vi "test Unsigned Integer Data Integrity.vi"(8 "error in (no error)":errorcluster, 11 "Data Manipulation Tests in":refnum<class "Data Manipulation Tests.lvclass">) -> (0 "error out":errorcluster, 3 "Data Manipulation Tests out":refnum<class "Data Manipulation Tests.lvclass">)   [LabVIEW 2017, in "Memory Manager Tests.lvlib" / "Data Manipulation Tests.lvclass"]
uses:
  Data Manipulation Tests.lvclass
  Source/Classes/Pointer/Write U8.vi
  Source/Classes/Pointer/Write U16.vi
  Source/Classes/Pointer/Write U32.vi
  Source/Classes/Pointer/Write U64.vi
  Source/Classes/Pointer/Write 1D U8.vi
  Source/Classes/Pointer/Write 1D U16.vi
  Source/Classes/Pointer/Write 1D U32.vi
  Source/Classes/Pointer/Write 1D U64.vi
  Source/Classes/Pointer/Pointer.lvclass
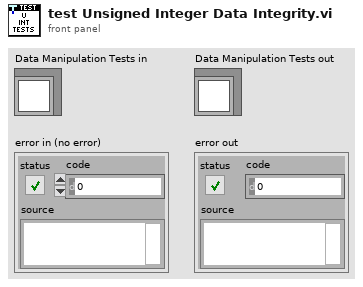
[diagram p1: front panel]
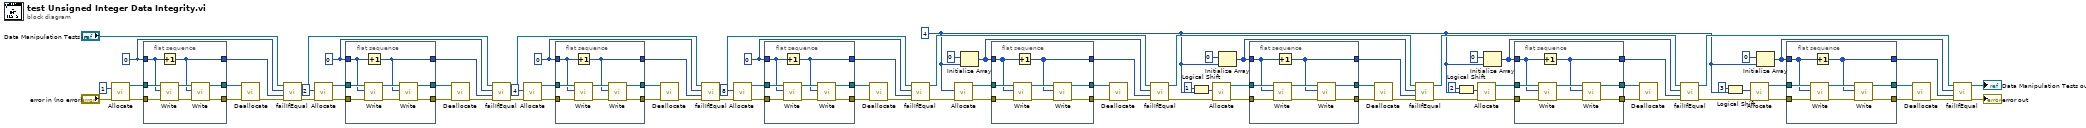
[diagram p0: block diagram]
diagram:
  w2 = u64 4 ("count (1)")
  w74 = u64 0 ("value")
  w84 = u32 0 ("value")
  w67 = u16 0 ("value")
  w56 = u8 0 ("value")
  n1 = call "Allocate.vi"("error in (no error)"="error in (no error)", "size"=u64 1) -> ("error out"=w58:errorcluster, "Pointer out"=w61:refnum<class "Pointer.lvclass">)  [unwired: 8 in]
  n2 = flat-sequence {
    tunnel: w61 -> [w97]
    tunnel: [w95] -> w60
    tunnel: [w94] -> w59
    tunnel: w58 -> [w92]
    tunnel: w56 -> [w91]
    tunnel: [w90] -> w55
    frame #0 {
      n3 = Increment(x=w91) -> (x+1=w90:u8)
      n4 = call-poly "Write.vi"("error in (no error)"=w92, "value"=w91, "Pointer in"=w97) -> ("error out"=w93:errorcluster, "Pointer out"=w96:refnum<class "Pointer.lvclass">)  [unwired: 5 in, 2 out]
      n5 = call-poly "Write.vi"("error in (no error)"=w93, "value"=w90, "Pointer in"=w96) -> ("error out"=w94:errorcluster, "Pointer out"=w95:refnum<class "Pointer.lvclass">)  [unwired: 5 in, 2 out]
    }
  }
  n6 = call "Deallocate.vi"("error in (no error)"=w59, "Pointer"=w60) -> ("error out"=w57:errorcluster)  [unwired: 8 in, 1 out]
  n7 = call-dynamic "failIfEqual.vi"("error in (no error)"=w57, "y"=w55, "x"=w56, "TestCase in"="Data Manipulation Tests in") -> ("error out"=w70:errorcluster, "TestCase out"=w69:refnum<class "Data Manipulation Tests.lvclass">)  [unwired: 6 in]
  n8 = call "Allocate.vi"("error in (no error)"=w70, "size"=u64 2) -> ("error out"=w65:errorcluster, "Pointer out"=w62:refnum<class "Pointer.lvclass">)  [unwired: 8 in]
  n9 = flat-sequence {
    tunnel: w62 -> [w105]
    tunnel: [w103] -> w63
    tunnel: [w102] -> w64
    tunnel: w65 -> [w100]
    tunnel: w67 -> [w99]
    tunnel: [w98] -> w68
    frame #0 {
      n10 = call-poly "Write.vi"("error in (no error)"=w100, "value"=w99, "Pointer in"=w105) -> ("error out"=w101:errorcluster, "Pointer out"=w104:refnum<class "Pointer.lvclass">)  [unwired: 5 in, 2 out]
      n11 = Increment(x=w99) -> (x+1=w98:u16)
      n12 = call-poly "Write.vi"("error in (no error)"=w101, "value"=w98, "Pointer in"=w104) -> ("error out"=w102:errorcluster, "Pointer out"=w103:refnum<class "Pointer.lvclass">)  [unwired: 5 in, 2 out]
    }
  }
  n13 = call "Deallocate.vi"("error in (no error)"=w64, "Pointer"=w63) -> ("error out"=w66:errorcluster)  [unwired: 8 in, 1 out]
  n14 = call-dynamic "failIfEqual.vi"("error in (no error)"=w66, "y"=w68, "x"=w67, "TestCase in"=w69) -> ("error out"=w87:errorcluster, "TestCase out"=w86:refnum<class "Data Manipulation Tests.lvclass">)  [unwired: 6 in]
  n15 = call "Allocate.vi"("error in (no error)"=w87, "size"=u64 4) -> ("error out"=w83:errorcluster, "Pointer out"=w80:refnum<class "Pointer.lvclass">)  [unwired: 8 in]
  n16 = flat-sequence {
    tunnel: w80 -> [w113]
    tunnel: [w111] -> w81
    tunnel: [w110] -> w82
    tunnel: w83 -> [w108]
    tunnel: w84 -> [w107]
    tunnel: [w106] -> w85
    frame #0 {
      n17 = call-poly "Write.vi"("error in (no error)"=w108, "value"=w107, "Pointer in"=w113) -> ("error out"=w109:errorcluster, "Pointer out"=w112:refnum<class "Pointer.lvclass">)  [unwired: 5 in, 2 out]
      n18 = Increment(x=w107) -> (x+1=w106:u32)
      n19 = call-poly "Write.vi"("error in (no error)"=w109, "value"=w106, "Pointer in"=w112) -> ("error out"=w110:errorcluster, "Pointer out"=w111:refnum<class "Pointer.lvclass">)  [unwired: 5 in, 2 out]
    }
  }
  n20 = call "Deallocate.vi"("error in (no error)"=w82, "Pointer"=w81) -> ("error out"=w9:errorcluster)  [unwired: 8 in, 1 out]
  n21 = call-dynamic "failIfEqual.vi"("error in (no error)"=w9, "y"=w85, "x"=w84, "TestCase in"=w86) -> ("error out"=w71:errorcluster, "TestCase out"=w72:refnum<class "Data Manipulation Tests.lvclass">)  [unwired: 6 in]
  n22 = call "Allocate.vi"("error in (no error)"=w71, "size"=u64 8) -> ("error out"=w76:errorcluster, "Pointer out"=w79:refnum<class "Pointer.lvclass">)  [unwired: 8 in]
  n23 = flat-sequence {
    tunnel: w79 -> [w121]
    tunnel: [w119] -> w78
    tunnel: [w118] -> w77
    tunnel: w76 -> [w116]
    tunnel: w74 -> [w115]
    tunnel: [w114] -> w73
    frame #0 {
      n24 = call-poly "Write.vi"("error in (no error)"=w116, "value"=w115, "Pointer in"=w121) -> ("error out"=w117:errorcluster, "Pointer out"=w120:refnum<class "Pointer.lvclass">)  [unwired: 5 in, 2 out]
      n25 = Increment(x=w115) -> (x+1=w114:u64)
      n26 = call-poly "Write.vi"("error in (no error)"=w117, "value"=w114, "Pointer in"=w120) -> ("error out"=w118:errorcluster, "Pointer out"=w119:refnum<class "Pointer.lvclass">)  [unwired: 5 in, 2 out]
    }
  }
  n27 = call "Deallocate.vi"("error in (no error)"=w77, "Pointer"=w78) -> ("error out"=w75:errorcluster)  [unwired: 8 in, 1 out]
  n28 = call-dynamic "failIfEqual.vi"("error in (no error)"=w75, "y"=w73, "x"=w74, "TestCase in"=w72) -> ("error out"=w24:errorcluster, "TestCase out"=w25:refnum<class "Data Manipulation Tests.lvclass">)  [unwired: 6 in]
  n29 = call "Allocate.vi"("error in (no error)"=w24, "size"=w2) -> ("error out"=w52:errorcluster, "Pointer out"=w49:refnum<class "Pointer.lvclass">)  [unwired: 8 in]
  n30 = Initialize Array(u8 0 ("value"), w2) -> (w20:u8[])
  n31 = flat-sequence {
    tunnel: w49 -> [w129]
    tunnel: [w127] -> w50
    tunnel: [w126] -> w51
    tunnel: w52 -> [w124]
    tunnel: w20 -> [w123]
    tunnel: [w122] -> w54
    frame #0 {
      n32 = call-poly "Write.vi"("error in (no error)"=w124, "buffer in"=w123, "Pointer in"=w129) -> ("error out"=w125:errorcluster, "Pointer out"=w128:refnum<class "Pointer.lvclass">)  [unwired: 5 in, 2 out]
      n33 = Increment(x=w123) -> (x+1=w122:u8[])
      n34 = call-poly "Write.vi"("error in (no error)"=w125, "buffer in"=w122, "Pointer in"=w128) -> ("error out"=w126:errorcluster, "Pointer out"=w127:refnum<class "Pointer.lvclass">)  [unwired: 5 in, 2 out]
    }
  }
  n35 = call "Deallocate.vi"("error in (no error)"=w51, "Pointer"=w50) -> ("error out"=w53:errorcluster)  [unwired: 8 in, 1 out]
  n36 = call-dynamic "failIfEqual.vi"("error in (no error)"=w53, "y"=w54, "x"=w20, "TestCase in"=w25) -> ("error out"=w41:errorcluster, "TestCase out"=w42:refnum<class "Data Manipulation Tests.lvclass">)  [unwired: 6 in]
  n37 = Logical Shift(y=i16 1, x=w2) -> (x << y=w8:u64)
  n38 = call "Allocate.vi"("error in (no error)"=w41, "size"=w8) -> ("error out"=w45:errorcluster, "Pointer out"=w48:refnum<class "Pointer.lvclass">)  [unwired: 8 in]
  n39 = Initialize Array(u16 0 ("value"), w2) -> (w18:u16[])
  n40 = flat-sequence {
    tunnel: w48 -> [w137]
    tunnel: [w135] -> w47
    tunnel: [w134] -> w46
    tunnel: w45 -> [w132]
    tunnel: w18 -> [w131]
    tunnel: [w130] -> w43
    frame #0 {
      n41 = call-poly "Write.vi"("error in (no error)"=w132, "buffer in"=w131, "Pointer in"=w137) -> ("error out"=w133:errorcluster, "Pointer out"=w136:refnum<class "Pointer.lvclass">)  [unwired: 5 in, 2 out]
      n42 = Increment(x=w131) -> (x+1=w130:u16[])
      n43 = call-poly "Write.vi"("error in (no error)"=w133, "buffer in"=w130, "Pointer in"=w136) -> ("error out"=w134:errorcluster, "Pointer out"=w135:refnum<class "Pointer.lvclass">)  [unwired: 5 in, 2 out]
    }
  }
  n44 = call "Deallocate.vi"("error in (no error)"=w46, "Pointer"=w47) -> ("error out"=w44:errorcluster)  [unwired: 8 in, 1 out]
  n45 = call-dynamic "failIfEqual.vi"("error in (no error)"=w44, "y"=w43, "x"=w18, "TestCase in"=w42) -> ("error out"=w26:errorcluster, "TestCase out"=w27:refnum<class "Data Manipulation Tests.lvclass">)  [unwired: 6 in]
  n46 = Logical Shift(y=i16 2, x=w2) -> (x << y=w5:u64)
  n47 = call "Allocate.vi"("error in (no error)"=w26, "size"=w5) -> ("error out"=w30:errorcluster, "Pointer out"=w33:refnum<class "Pointer.lvclass">)  [unwired: 8 in]
  n48 = Initialize Array(u32 0 ("value"), w2) -> (w16:u32[])
  n49 = flat-sequence {
    tunnel: w33 -> [w145]
    tunnel: [w143] -> w32
    tunnel: [w142] -> w31
    tunnel: w30 -> [w140]
    tunnel: w16 -> [w139]
    tunnel: [w138] -> w28
    frame #0 {
      n50 = call-poly "Write.vi"("error in (no error)"=w140, "buffer in"=w139, "Pointer in"=w145) -> ("error out"=w141:errorcluster, "Pointer out"=w144:refnum<class "Pointer.lvclass">)  [unwired: 5 in, 2 out]
      n51 = Increment(x=w139) -> (x+1=w138:u32[])
      n52 = call-poly "Write.vi"("error in (no error)"=w141, "buffer in"=w138, "Pointer in"=w144) -> ("error out"=w142:errorcluster, "Pointer out"=w143:refnum<class "Pointer.lvclass">)  [unwired: 5 in, 2 out]
    }
  }
  n53 = call "Deallocate.vi"("error in (no error)"=w31, "Pointer"=w32) -> ("error out"=w29:errorcluster)  [unwired: 8 in, 1 out]
  n54 = call-dynamic "failIfEqual.vi"("error in (no error)"=w29, "y"=w28, "x"=w16, "TestCase in"=w27) -> ("error out"=w3:errorcluster, "TestCase out"=w40:refnum<class "Data Manipulation Tests.lvclass">)  [unwired: 6 in]
  n55 = Logical Shift(y=i16 3, x=w2) -> (x << y=w1:u64)
  n56 = call "Allocate.vi"("error in (no error)"=w3, "size"=w1) -> ("error out"=w37:errorcluster, "Pointer out"=w34:refnum<class "Pointer.lvclass">)  [unwired: 8 in]
  n57 = Initialize Array(u64 0 ("value"), w2) -> (w14:u64[])
  n58 = flat-sequence {
    tunnel: w34 -> [w153]
    tunnel: [w151] -> w35
    tunnel: [w150] -> w36
    tunnel: w37 -> [w148]
    tunnel: w14 -> [w147]
    tunnel: [w146] -> w39
    frame #0 {
      n59 = call-poly "Write.vi"("error in (no error)"=w148, "buffer in"=w147, "Pointer in"=w153) -> ("error out"=w149:errorcluster, "Pointer out"=w152:refnum<class "Pointer.lvclass">)  [unwired: 5 in, 2 out]
      n60 = Increment(x=w147) -> (x+1=w146:u64[])
      n61 = call-poly "Write.vi"("error in (no error)"=w149, "buffer in"=w146, "Pointer in"=w152) -> ("error out"=w150:errorcluster, "Pointer out"=w151:refnum<class "Pointer.lvclass">)  [unwired: 5 in, 2 out]
    }
  }
  n62 = call "Deallocate.vi"("error in (no error)"=w36, "Pointer"=w35) -> ("error out"=w38:errorcluster)  [unwired: 8 in, 1 out]
  n63 = call-dynamic "failIfEqual.vi"("error in (no error)"=w38, "y"=w39, "x"=w14, "TestCase in"=w40) -> ("error out"=→"error out":errorcluster, "TestCase out"=→"Data Manipulation Tests out":refnum<class "Data Manipulation Tests.lvclass">)  [unwired: 6 in]
